vi "SaveResults.vi"(8 "error in (no error)":errorcluster, 10 "AcLoad":refnum<class "AcPwrBase.lvclass">, 11 "AcSave in":refnum<class "AcPwrBase.lvclass">) -> (0 "error out":errorcluster, 3 "AcSave out":refnum<class "AcPwrBase.lvclass">)   [LabVIEW 2018, in "AcPwrPlugins.lvlib" / "AcPwrBase.lvclass"]
uses:
  AcPwrBase.lvclass
  AcPwrBase.lvclass/AcPwrBase.ctl
  Accessors/Read BaseMeasures.vi
  Accessors/Write BaseMeasures.vi
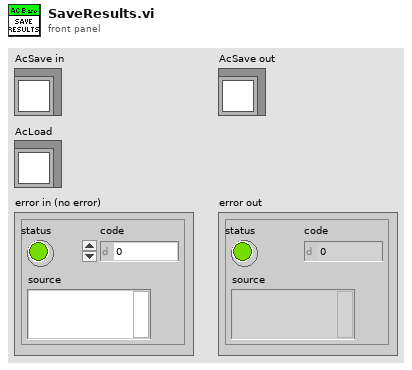
[diagram p1: front panel]
types:
  T1 = typedef "AcPwrPlugins.lvlib/AcPwrBase.lvclass/BaseMeasure.ctl" = cluster{"Handle":string, "Name":string, "Enabled":bool, "Result":dbl, "MeasType":T2, "btnMeasFetch":bool, "Hold Peak?":bool}
  T2 = typedef "AcPwrPlugins.lvlib/AcPwrBase.lvclass/MeasType.ctl" = enum16{"Voltage RMS L-N", "Current RMS", "Frequency", "Voltage DC", "Current DC", "Power Factor", "Current Peak", "Power VA", "Real Power", "Voltage THD", "Voltage EHD", "Voltage OHD", "Current THD", "Current EHD", "Current OHD", "Voltage RMS L-L", "Phase Angle", "Power DC", "Crest Factor"}
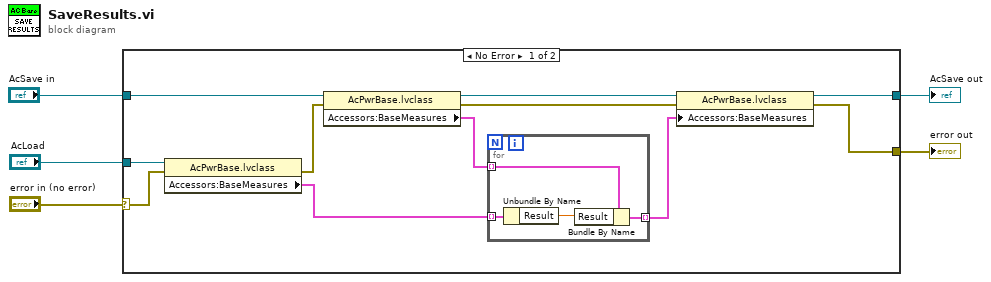
[diagram p0: block diagram]
diagram:
  n1 = case shown="No Error" "error in (no error)" {
    selector: "error in (no error)" -> [w9 w22]
    tunnel: [w16 w21] -> w5
    tunnel: "AcLoad" -> [w14 _]
    tunnel: [w10 w22] -> w3
    tunnel: "AcSave in" -> [w6 w21]
    frame No Error {
      n2 = property class="AcPwrBase.lvclass"(reference=w14, error in=w9) -> (error out=w8:errorcluster, "Accessors:BaseMeasures"=w13:T1[])  [unwired: 1 out]
      n3 = property class="AcPwrBase.lvclass"(reference=w6, error in=w8) -> (reference out=w12:refnum<class "AcPwrBase.lvclass">, error out=w7:errorcluster, "Accessors:BaseMeasures"=w15:T1[])
      n4 = for {
        tunnel: w15 -> [w18] mode=indexing
        tunnel: w13 -> [w19] mode=indexing
        tunnel: [w17] -> w11 mode=indexing
        n5 = Unbundle By Name(w19) -> ("Result"=w20:dbl)
        n6 = Bundle By Name(cluster=w18, "Result"=w20) -> (w17:T1)
      }
      n7 = property class="AcPwrBase.lvclass"(reference=w12, error in=w7, "Accessors:BaseMeasures"=w11) -> (reference out=w16:refnum<class "AcPwrBase.lvclass">, error out=w10:errorcluster)
    }
    frame Error {
    }
  }
  "error out" <- w3
  "AcSave out" <- w5
